vi "BioFeedback18(Producer+Consumer).vi"() -> ()   [LabVIEW 2016]
doc: "Use this template to build a producer/consumer design pattern. Use this template when you need to execute a process, such as data analysis, when a data source, such as a triggered acquisition, produces data at an uneven rate and you need to execute the process when the data becomes available."
uses:
  customSubVIs/8ChanWfmArray.ctl
  <vilib>/Waveform/WDTFileIO.llb/Export Waveforms To Spreadsheet File (1D).vi
panel:
  out "Disp Data":cluster{"queue out":refnum<queue>, dbl, dbl}[](array[cluster])
  in  "Target Percentage":dbl=10.0
  out "DisplayActivation":dbl
  out "DisplayBarActivation":dbl(slide) caption="Left" max=1.0 scale=0.0..100.0
  in  "Display Channel":dbl=0.5
  out "MVC Data":cluster{"queue out":refnum<queue>, dbl, dbl}[](array[cluster])
  in  "Base Name":string="Test"
  in  "Data Directory":path=path "C:/Users/Tinggroup/Desktop/VRMuscleActivationVisualizer/LabviewFiles/Data/Test"
  out "GetMaxStartTime":timestamp
  in  "MVC Number":dbl=1.0
  in  "SecondsToAcquireMax":dbl=3.0
  in  "Frames Per Second":dbl=30.0 caption="Upper Cut-Off"
  in  "EMG Input Device\nProduct Type":string="USB-6009"
  out "raw data":dynamicdata(graph)
  out "dispSize":dbl=20.0 caption="Lower Cut-Off"
  out "mvcSize":dbl=300.0 caption="Upper Cut-Off"
  in  "MVC Window Size (s)":dbl=0.5
  in  "Display Window Size (s)":dbl=0.5
  in  "MVC Raw Path":path
  in  "trial raw data":path
  in  "trial filtered data":path
  in  "MVC Filtered Path":path
  in  "Sample rate (Hz)":dbl=1000.0 caption="Upper Cut-Off"
  out "fps":dbl=20.0 caption="Lower Cut-Off"
  out "rate":dbl=300.0 caption="Upper Cut-Off"
  in  "Set Parameters":bool
  out "lower":dbl=20.0 caption="Lower Cut-Off"
  out "upper":dbl=300.0 caption="Upper Cut-Off"
  in  "Lower Cut-Off":dbl=20.0
  in  "Upper Cut-Off":dbl=500.0
  in  "Mark":bool
  in  "End Trial":bool
  in  "Reset MVC":bool
  in  "Get MVC":bool
  in  "StartTrial":bool
  out "State":T1(ring)
  out "FilteredAndRectified":waveform(dbl)[](graph) caption="Filtered and Rectified"
  in  "stop":bool
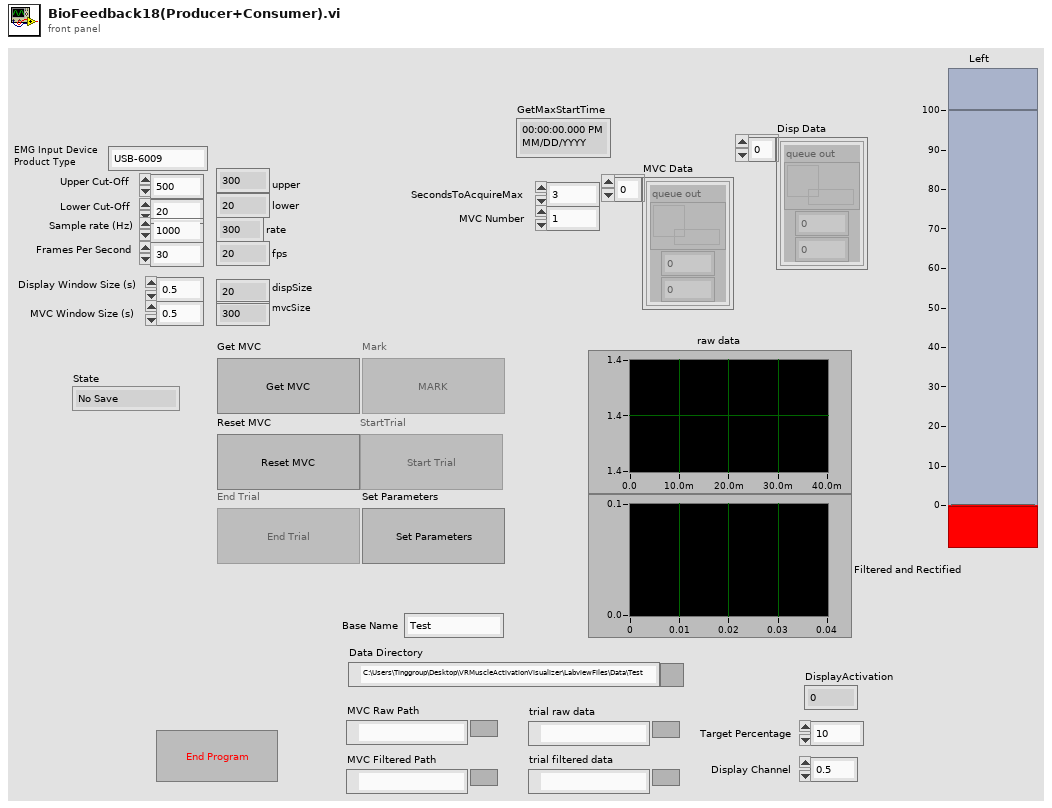
[diagram p1: front panel]
types:
  T1 = enum16{"No Save", "Acquiring Max", "Trial In Progress"}
  T2 = typedef "8ChanWfmArray.ctl" = waveform(dbl)[]
  T3 = enum8{"Enabled", "Disabled", "Disabled and Grayed Out"}
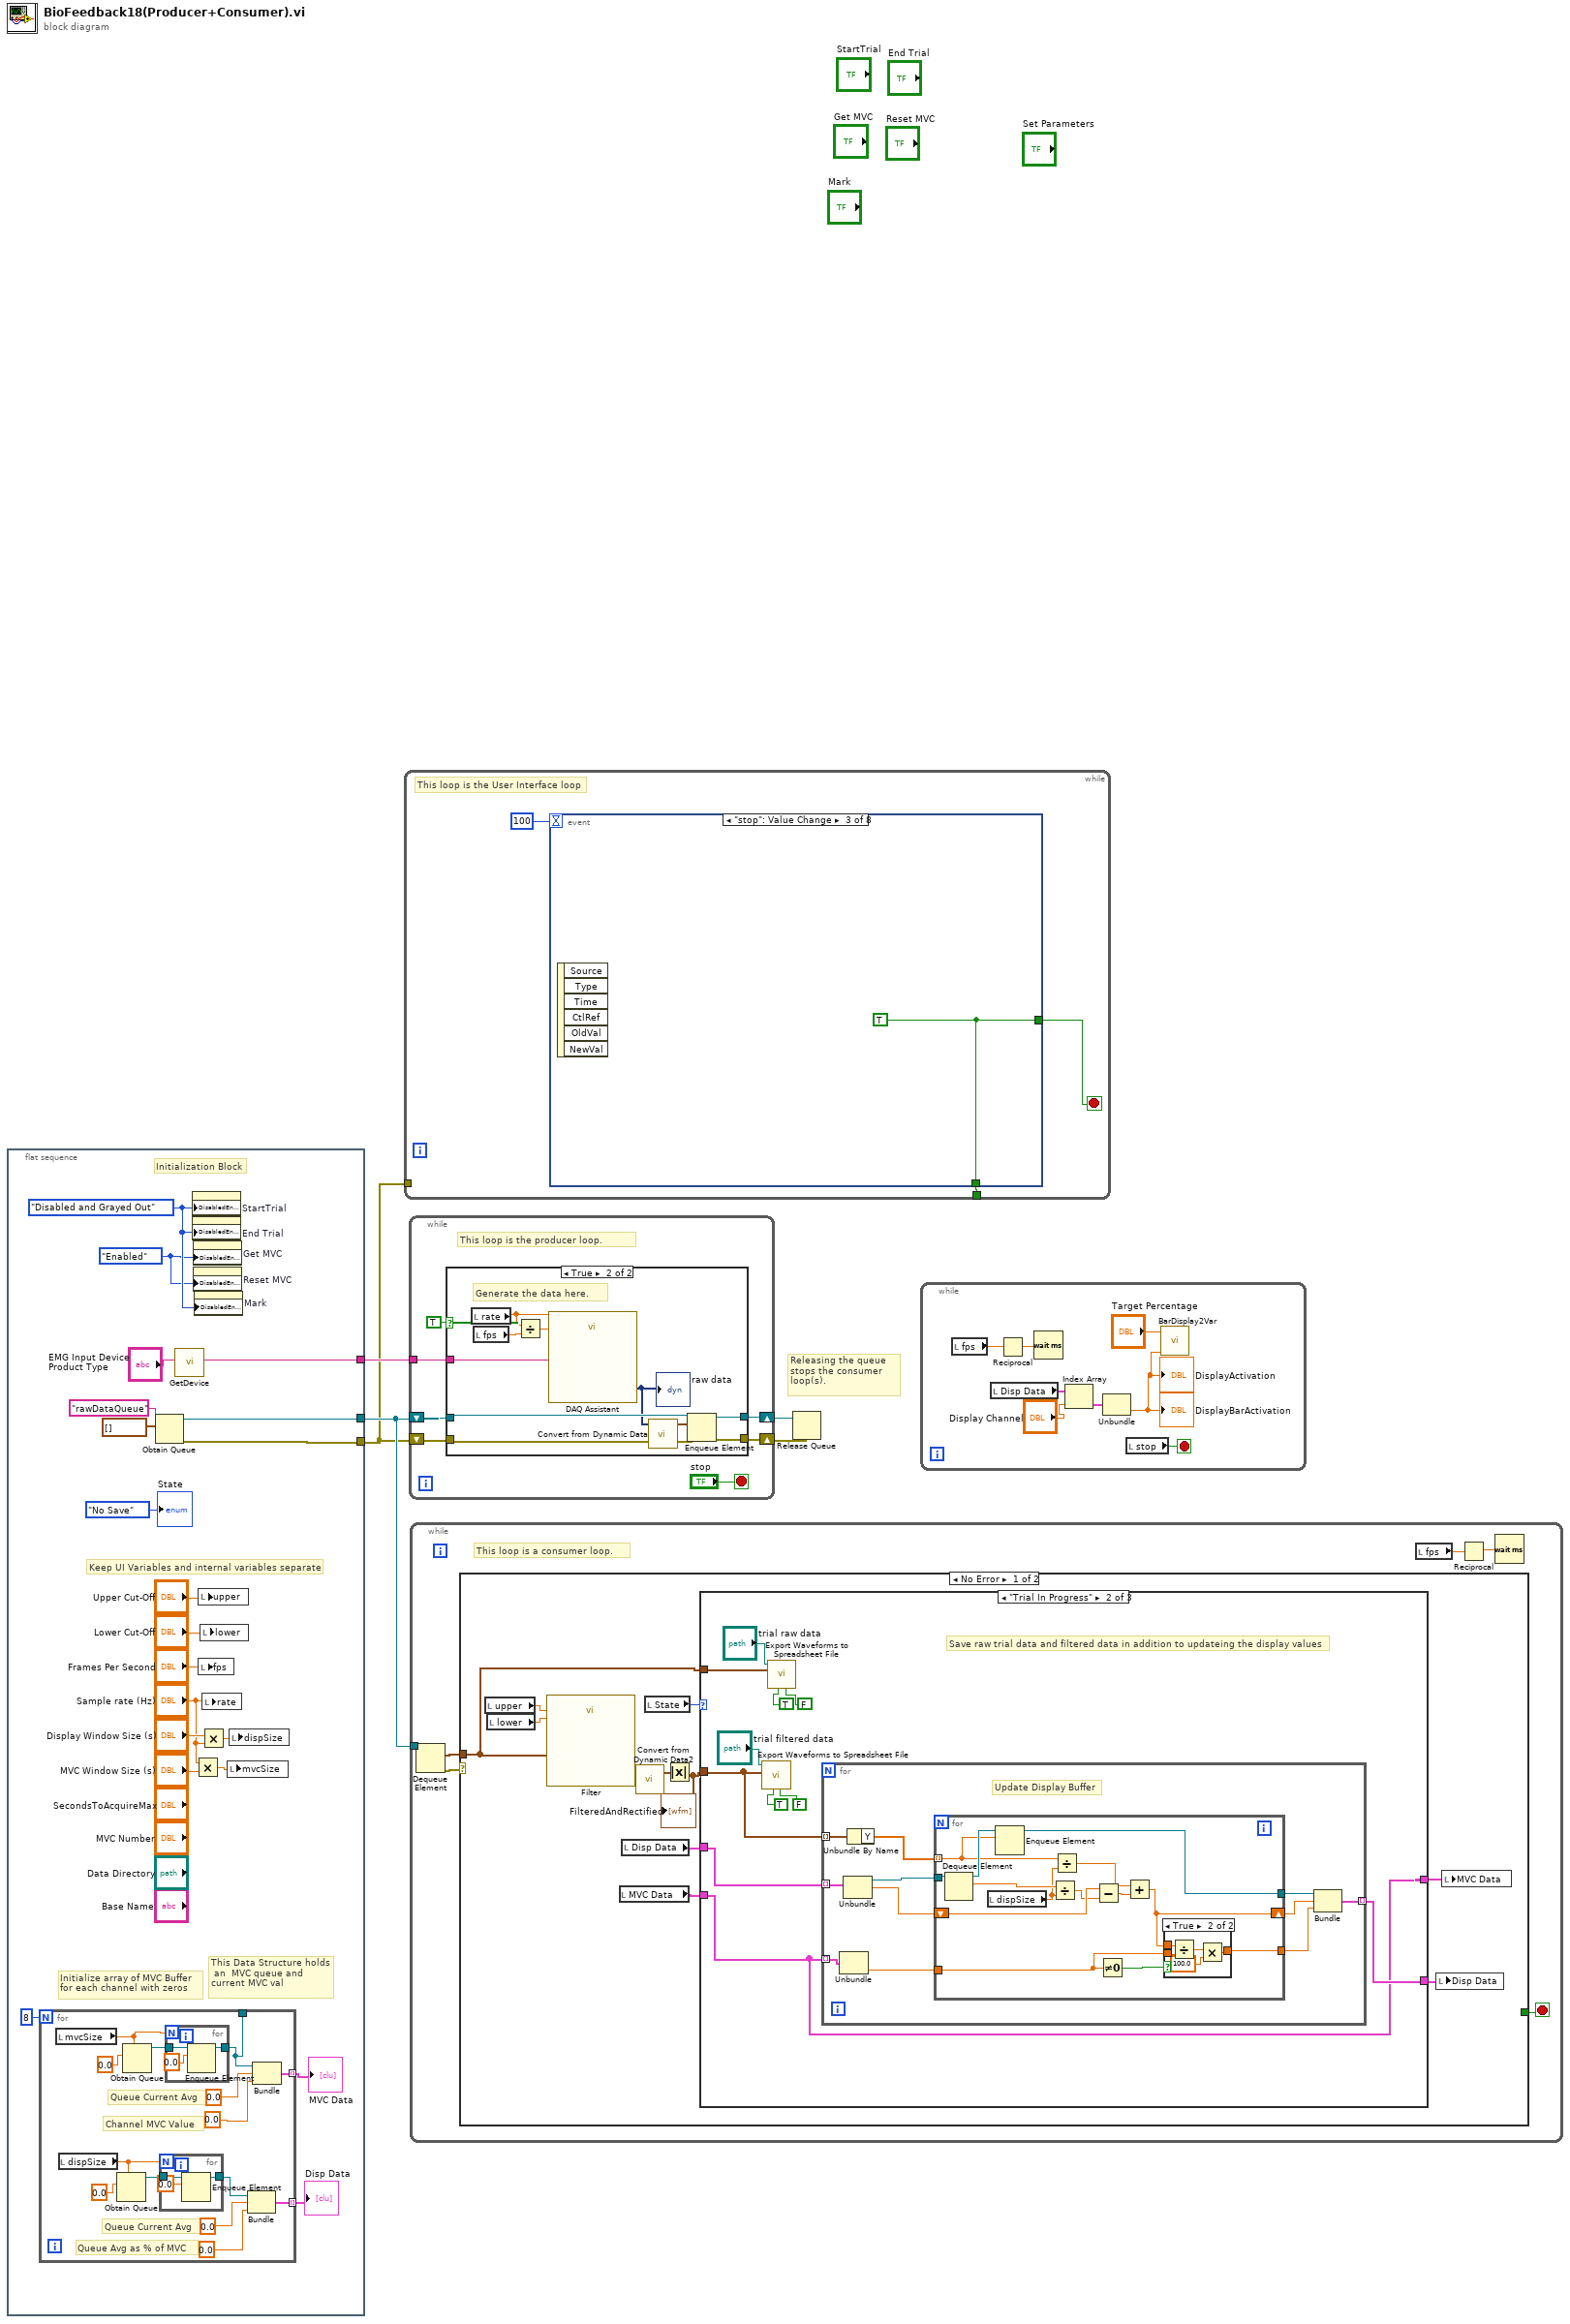
[diagram p0: block diagram]
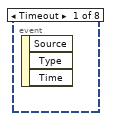
[diagram p2: hidden frame]
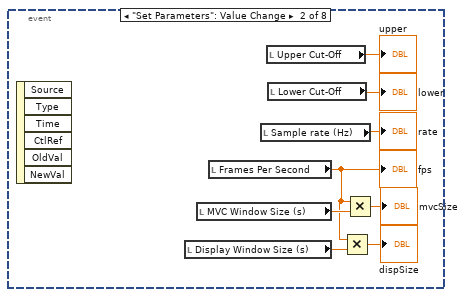
[diagram p3: hidden frame]
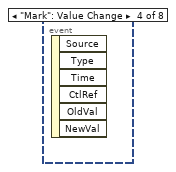
[diagram p4: hidden frame]
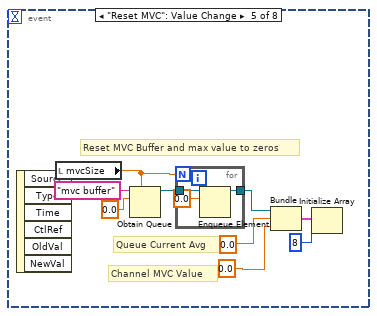
[diagram p5: hidden frame]
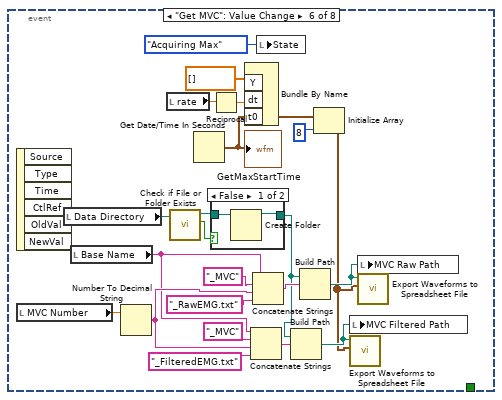
[diagram p6: hidden frame]
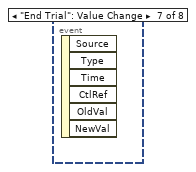
[diagram p8: hidden frame]
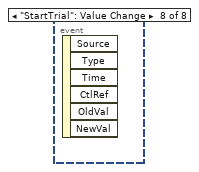
[diagram p9: hidden frame]
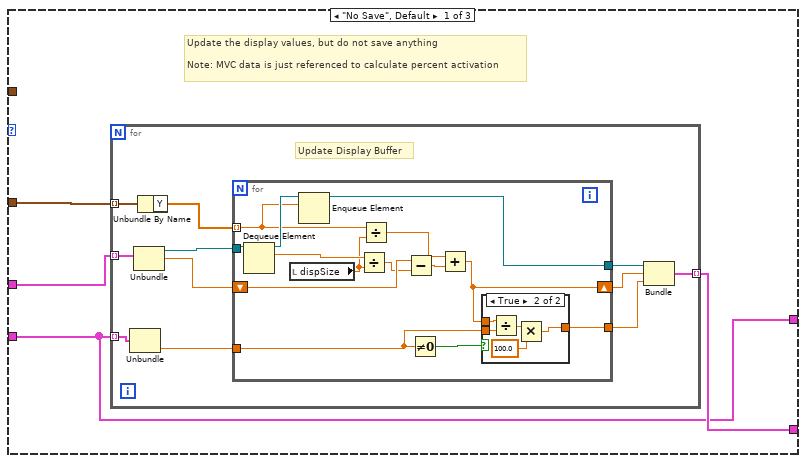
[diagram p10: hidden frame]
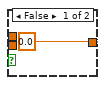
[diagram p11: hidden frame]
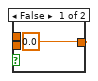
[diagram p12: hidden frame]
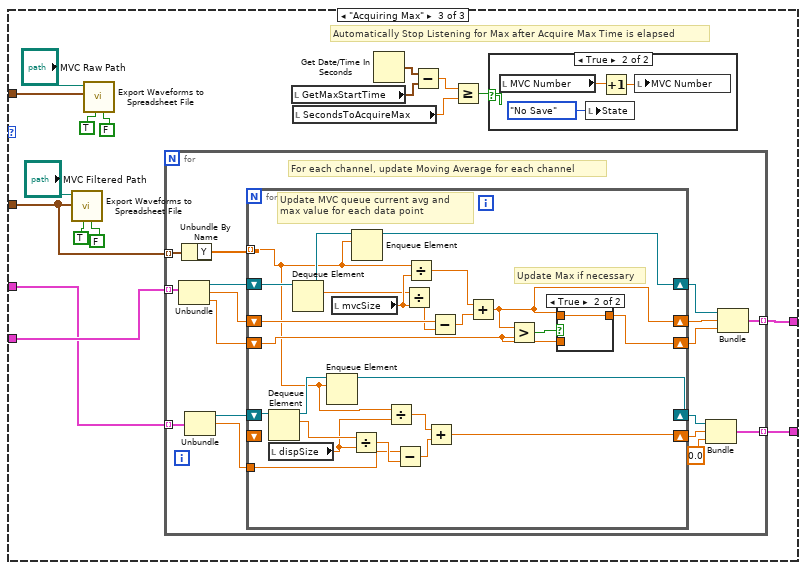
[diagram p13: hidden frame]
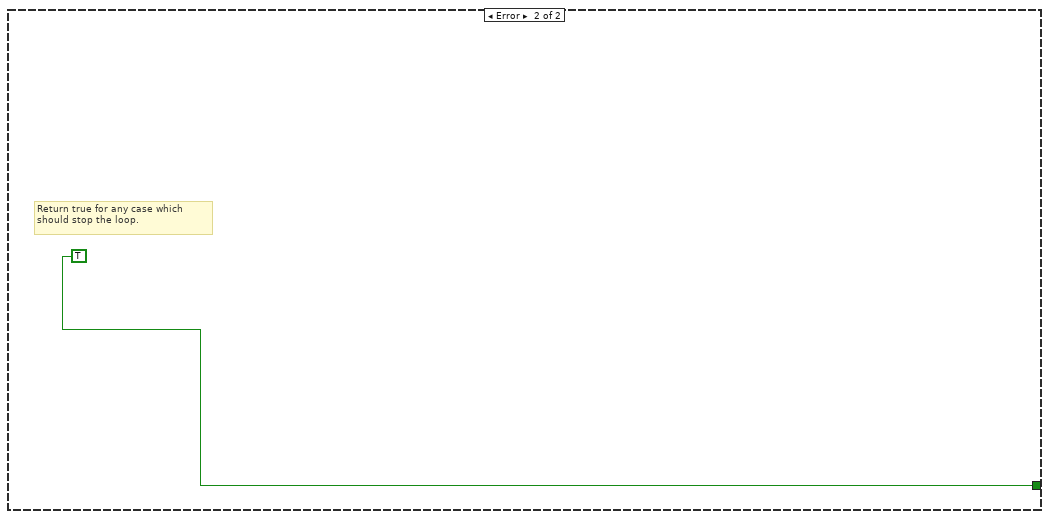
[diagram p16: hidden frame]
diagram:
  # "Releasing the queue stops the consumer loop(s)."
  n1 = flat-sequence {
    tunnel: [w16] -> w2
    tunnel: [w15] -> w1
    tunnel: [w18] -> w3
    frame #0 {
      w22 = T3."Enabled" ("Disabled")
      w23 = T3."Disabled and Grayed Out" ("Disabled")
      # "Keep UI Variables and internal variables separate"
      # "This Data Structure holds\n an  MVC queue and \ncurrent MVC val"
      # "Initialize array of MVC Buffer \nfor each channel with zeros"
      # "Initialization Block"
      n2 = for {
        N: 8 -> [_]
        tunnel: [w36] -> w8 mode=indexing
        tunnel: [w33] -> _
        tunnel: [w26] -> w7 mode=indexing
        # "Queue Avg as % of MVC"
        # "Queue Current Avg"
        # "Channel MVC Value"
        # "Queue Current Avg"
        n3 = local read "mvcSize"() -> (w37:dbl)
        n4 = local read "dispSize"() -> (w30:dbl)
        n5 = Obtain Queue(max queue size (-1, unlimited)=w30, element data type=0.0) -> (queue out=w27:refnum<queue>)  [unwired: 3 in, 2 out]
        n6 = Obtain Queue(max queue size (-1, unlimited)=w37, element data type=0.0) -> (queue out=w38:refnum<queue>)  [unwired: 3 in, 2 out]
        n7 = for {
          N: w30 -> [_]
          tunnel: w27 -> [w42]
          tunnel: [w40] -> w28
          n8 = Enqueue Element(queue=w42, element=0.0) -> (queue out=w40:refnum<queue>)  [unwired: 2 in, 2 out]
        }
        n9 = for {
          N: w37 -> [_]
          tunnel: w38 -> [w45]
          tunnel: [w43] -> w33
          n10 = Enqueue Element(queue=w45, element=0.0) -> (queue out=w43:refnum<queue>)  [unwired: 2 in, 2 out]
        }
        n11 = Bundle("queue out"=w28, 0.0, 0.0) -> (w26:cluster{"queue out":refnum<queue>, dbl, dbl})  [unwired: 1 in]
        n12 = Bundle("queue out"=w33, 0.0, 0.0) -> (w36:cluster{"queue out":refnum<queue>, dbl, dbl})  [unwired: 1 in]
      }
      "MVC Data" <- w8
      "Disp Data" <- w7
      n13 = Obtain Queue(name (unnamed)="rawDataQueue", element data type=T2 [] ("initialized array")) -> (queue out=w16:refnum<queue>, error out=w15:errorcluster)  [unwired: 3 in, 1 out]
      n14 = call "GetDevice.vi"("EMG Input Device\nProduct Type"="EMG Input Device\nProduct Type") -> ("DAQmx Device Name"=w18:tag)  [unwired: 10 in]
      n15 = property on="StartTrial" class="Bool"("DisabledEnum"=w23) -> ()  [unwired: 2 in, 2 out]
      n16 = property on="End Trial" class="Bool"("DisabledEnum"=w23) -> ()  [unwired: 2 in, 2 out]
      n17 = property on="Get MVC" class="Bool"("DisabledEnum"=w22) -> ()  [unwired: 2 in, 2 out]
      n18 = property on="Reset MVC" class="Bool"("DisabledEnum"=w22) -> ()  [unwired: 2 in, 2 out]
      n19 = property on="Mark" class="Bool"("DisabledEnum"=w23) -> ()  [unwired: 2 in, 2 out]
      n20 = Multiply(x="Sample rate (Hz)", y="MVC Window Size (s)") -> (x*y=w10:dbl)
      n21 = local write "upper"("Upper Cut-Off") -> ()
      n22 = local write "fps"("Frames Per Second") -> ()
      n23 = Multiply(x="Display Window Size (s)", y="Sample rate (Hz)") -> (x*y=w13:dbl)
      n24 = local write "lower"("Lower Cut-Off") -> ()
      n25 = local write "rate"("Sample rate (Hz)") -> ()
      n26 = local write "mvcSize"(w10) -> ()
      n27 = local write "dispSize"(w13) -> ()
      "State" <- T1."No Save" ("State")
    }
  }
  n28 = while {
    tunnel: [w47] -> _
    tunnel: w1 -> [_]
    stop <- w48 stop-if-true
    # "This loop is the User Interface loop"
    n29 = event shown="[2] \"stop\": Value Change" {
      selector: _ -> [_ _ _ _ _ _ _ _]
      dyn-events: _ -> [_ _ _ _ _ _ _ _]
      timeout: u32 100 ("milliseconds to wait") -> [_ _ _ _ _ _ _ _]
      tunnel: [_ _ w57 _ _ _ _ _] -> w48
      tunnel: [_ _ w57 _ _ _ _ _] -> w47
      event Timeout {
        n30 = event-data() -> ()  [unwired: 1 in, 3 out]
      }
      event "Set Parameters": Value Change {
        n31 = event-data() -> ()  [unwired: 1 in, 6 out]
        n32 = local read "Display Window Size (s)"() -> (w52:dbl)
        n33 = local read "MVC Window Size (s)"() -> (w53:dbl)
        n34 = local read "Frames Per Second"() -> (w51:dbl)
        "fps" <- w51
        n35 = local read "Sample rate (Hz)"() -> (→"rate":dbl)
        n36 = local read "Upper Cut-Off"() -> (→"upper":dbl)
        n37 = local read "Lower Cut-Off"() -> (→"lower":dbl)
        n38 = Multiply(x=w51, y=w52) -> (x*y=→"dispSize":dbl)
        n39 = Multiply(x=w51, y=w53) -> (x*y=→"mvcSize":dbl)
      }
      event "stop": Value Change {
        w57 = TRUE
        n40 = event-data() -> ()  [unwired: 1 in, 6 out]
      }
      event "Mark": Value Change {
        n41 = event-data() -> ()  [unwired: 1 in, 6 out]
      }
      event "Reset MVC": Value Change {
        # "Channel MVC Value"
        # "Queue Current Avg"
        # "Reset MVC Buffer and max value to zeros"
        n42 = event-data() -> ()  [unwired: 1 in, 6 out]
        n43 = local read "mvcSize"() -> (w61:dbl)
        n44 = Obtain Queue(max queue size (-1, unlimited)=w61, name (unnamed)="mvc buffer", element data type=0.0) -> (queue out=w60:refnum<queue>)  [unwired: 2 in, 2 out]
        n45 = for {
          N: w61 -> [_]
          tunnel: w60 -> [w69]
          tunnel: [w67] -> w63
          n46 = Enqueue Element(queue=w69, element=0.0) -> (queue out=w67:refnum<queue>)  [unwired: 2 in, 2 out]
        }
        n47 = Bundle("queue out"=w63, 0.0, 0.0) -> (w64:cluster{"queue out":refnum<queue>, dbl, dbl})  [unwired: 1 in]
        n48 = Initialize Array(w64, 8 ("dimension size")) -> ()  [unwired: 1 out]
      }
      event "Get MVC": Value Change {
        n49 = event-data() -> ()  [unwired: 1 in, 6 out]
        n50 = local read "MVC Number"() -> (w79:dbl)
        n51 = local read "Data Directory"() -> (w80:path)
        n52 = local read "Base Name"() -> (w77:string)
        n53 = Number To Decimal String(number=w79) -> (decimal integer string=w78:string)  [unwired: 1 in]
        n54 = local read "rate"() -> (w74:dbl)
        n55 = call <vilib>:"Check if File or Folder Exists.vi"("path"=w80) -> ("file or folder exists?"=w82:bool, "dup path"=w81:path)  [unwired: 8 in, 1 out]
        n56 = Get Date/Time In Seconds() -> (seconds since 1Jan1904=w70:timestamp)
        "GetMaxStartTime" <- w70
        n57 = Reciprocal(x=w74) -> (1/x=w73:dbl)
        n58 = case shown="False" w82 {
          tunnel: w81 -> [w94 w95]
          tunnel: [w93 w95] -> w83
          frame False {
            n59 = Create Folder(path (use dialog)=w94) -> (created path=w93:path)  [unwired: 2 in, 2 out]
          }
          frame True {
          }
        }
        n60 = Bundle By Name("Y"=dbl[] [], "dt"=w73, "t0"=w70) -> (w76:waveform(dbl))  [unwired: 1 in]
        n61 = Concatenate Strings(w77, "_MVC" ("string"), w78, "_FilteredEMG.txt" ("string")) -> (w90:string)
        n62 = Concatenate Strings(w77, "_MVC" ("string"), w78, "_RawEMG.txt" ("string")) -> (w89:string)
        n63 = local write "State"(T1."Acquiring Max" ("State")) -> ()
        n64 = Build Path(base path=w83, name or relative path=w90) -> (appended path=w84:path)
        n65 = Build Path(base path=w83, name or relative path=w89) -> (appended path=w85:path)
        n66 = Initialize Array(w76, 8 ("dimension size")) -> (w75:waveform(dbl)[])
        n67 = local write "MVC Filtered Path"(w84) -> ()
        n68 = call-poly <vilib>:"Export Waveforms to Spreadsheet File.vi"("waveforms"=w75, "file path (dialog if empty)"=w84) -> ()  [unwired: 8 in, 2 out]
        n69 = local write "MVC Raw Path"(w85) -> ()
        n70 = call-poly <vilib>:"Export Waveforms to Spreadsheet File.vi"("waveforms"=w75, "file path (dialog if empty)"=w85) -> ()  [unwired: 8 in, 2 out]
      }
      event "End Trial": Value Change {
        n71 = event-data() -> ()  [unwired: 1 in, 6 out]
      }
      event "StartTrial": Value Change {
        n72 = event-data() -> ()  [unwired: 1 in, 6 out]
      }
    }
  }
  n73 = while {
    shift-right: [w98] -> w4
    shift-left: w1 -> [w99]
    shift-right: [w100] -> w5
    shift-left: w2 -> [w101]
    tunnel: w3 -> [w96]
    stop <- "stop" stop-if-true
    # "This loop is the producer loop."
    n74 = case shown="True" TRUE ("Case Constant\n(See Context Help)") {
      tunnel: w101 -> [w104 w114]
      tunnel: [w104 w113] -> w100
      tunnel: w99 -> [w103 w112]
      tunnel: [w103 w111] -> w98
      tunnel: w96 -> [_ w105]
      frame False {
      }
      frame True {
        # "Generate the data here."
        n75 = local read "rate"() -> (w108:dbl)
        n76 = local read "fps"() -> (w109:dbl)
        n77 = Divide(x=w108, y=w109) -> (x/y=w107:dbl)
        n78 = call "DAQ Assistant"("rate"=w108, "number of samples"=w107, "device name"=w105) -> ("data"=w106:dynamicdata)  [unwired: 13 in, 3 out]
        "raw data" <- w106
        n79 = call "Convert from Dynamic Data"("Dynamic Data Type"=w106) -> ("Array of Waveform"=w110:waveform(dbl)[])  [unwired: 3 in]
        n80 = Enqueue Element(queue=w114, element=w110, error in (no error)=w112) -> (queue out=w113:refnum<queue>, error out=w111:errorcluster)  [unwired: 1 in, 1 out]
      }
    }
  }
  n81 = while {
    tunnel: w2 -> [w117]
    stop <- w118 stop-if-true
    # "This loop is a consumer loop."
    n82 = Dequeue Element(queue=w117) -> (element=w119:T2, error out=w120:errorcluster)  [unwired: 2 in, 2 out]
    n83 = case shown="No Error" w120 {
      tunnel: w119 -> [w126 _]
      tunnel: [_ TRUE] -> w118
      frame No Error {
        n84 = local read "upper"() -> (w129:dbl)
        n85 = local read "lower"() -> (w128:dbl)
        n86 = call "Filter"("Lower Cut-Off"=w128, "Upper Cut-Off"=w129, "Signal"=w126) -> ("Filtered Signal"=w130:dynamicdata)  [unwired: 7 in, 1 out]
        n87 = local read "MVC Data"() -> (w124:cluster{"queue out":refnum<queue>, dbl, dbl}[])
        n88 = local read "Disp Data"() -> (w123:cluster{"queue out":refnum<queue>, dbl, dbl}[])
        n89 = call "Convert from Dynamic Data2"("Dynamic Data Type"=w130) -> ("Array of Waveform"=w131:waveform(dbl)[])  [unwired: 3 in]
        n90 = local read "State"() -> (w127:T1)
        n91 = Absolute Value(x=w131) -> (abs(x)=w125:waveform(dbl)[])
        "FilteredAndRectified" <- w125
        n92 = case shown="\"Trial In Progress\"" w127 {
          tunnel: w125 -> [w135 w169 w219]
          tunnel: w126 -> [_ w172 w220]
          tunnel: w124 -> [w132 w167 w210]
          tunnel: w123 -> [w134 w170 w209]
          tunnel: [w133 w168 w211] -> w121
          tunnel: [w132 w167 w212] -> w122
          frame "No Save", Default {
            # "Update the display values, but do not save anything\n\nNote: MVC data is just referenced to calculate percent activation"
            n93 = for {
              tunnel: w134 -> [w140] mode=indexing
              tunnel: w135 -> [w145] mode=indexing
              tunnel: [w141] -> w133 mode=indexing
              tunnel: w132 -> [w138] mode=indexing
              # "Update Display Buffer"
              n94 = Unbundle(w138) -> (w137:dbl)  [unwired: 2 out]
              n95 = Unbundle(w140) -> ("queue out"=w146:refnum<queue>, w139:dbl)  [unwired: 1 out]
              n96 = Unbundle By Name(w145) -> ("Y"=w144:dbl[])
              n97 = for {
                tunnel: w146 -> [w154]
                tunnel: w144 -> [w150] mode=indexing
                shift-right: [w148] -> w143
                shift-left: w139 -> [w159]
                tunnel: [w149] -> w142
                tunnel: w137 -> [w152]
                tunnel: [w147] -> w136
                n98 = Dequeue Element(queue=w154) -> (queue out=w151:refnum<queue>, element=w160:dbl)  [unwired: 2 in, 2 out]
                n99 = local read "dispSize"() -> (w157:dbl)
                n100 = Enqueue Element(queue=w151, element=w150) -> (queue out=w149:refnum<queue>)  [unwired: 2 in, 2 out]
                n101 = Divide(x=w160, y=w157) -> (x/y=w158:dbl)
                n102 = Divide(x=w150, y=w157) -> (x/y=w155:dbl)
                n103 = Subtract(x=w159, y=w158) -> (x-y=w156:dbl)
                n104 = Not Equal To 0?(x=w152) -> (x != 0?=w153:bool)
                n105 = Add(x=w155, y=w156) -> (x+y=w148:dbl)
                n106 = case shown="True" w153 {
                  tunnel: w152 -> [_ w166]
                  tunnel: [0.0 w162] -> w147
                  tunnel: w148 -> [_ w165]
                  frame False {
                  }
                  frame True {
                    n107 = Divide(x=w165, y=w166) -> (x/y=w163:dbl)
                    n108 = Multiply(x=w163, y=100.0) -> (x*y=w162:dbl)
                  }
                }
              }
              n109 = Bundle("queue out"=w142, w143, w136) -> (w141:cluster{"queue out":refnum<queue>, dbl, dbl})  [unwired: 1 in]
            }
          }
          frame "Trial In Progress" {
            # "Save raw trial data and filtered data in addition to updateing the display values"
            n110 = call-poly <vilib>:"Export Waveforms to Spreadsheet File.vi"("header? (write header:T)"=FALSE, "append to file? (new file:F)"=TRUE, "waveforms"=w169, "file path (dialog if empty)"="trial filtered data") -> ()  [unwired: 6 in, 2 out]
            n111 = call-poly <vilib>:"Export Waveforms to Spreadsheet File.vi"("header? (write header:T)"=FALSE, "append to file? (new file:F)"=TRUE, "waveforms"=w172, "file path (dialog if empty)"="trial raw data") -> ()  [unwired: 6 in, 2 out]
            n112 = for {
              tunnel: w170 -> [w182] mode=indexing
              tunnel: w169 -> [w187] mode=indexing
              tunnel: [w183] -> w168 mode=indexing
              tunnel: w167 -> [w180] mode=indexing
              # "Update Display Buffer"
              n113 = Unbundle(w180) -> (w179:dbl)  [unwired: 2 out]
              n114 = Unbundle(w182) -> ("queue out"=w188:refnum<queue>, w181:dbl)  [unwired: 1 out]
              n115 = Unbundle By Name(w187) -> ("Y"=w186:dbl[])
              n116 = for {
                tunnel: w188 -> [w196]
                tunnel: w186 -> [w192] mode=indexing
                shift-right: [w190] -> w185
                shift-left: w181 -> [w201]
                tunnel: [w191] -> w184
                tunnel: w179 -> [w194]
                tunnel: [w189] -> w178
                n117 = Dequeue Element(queue=w196) -> (queue out=w193:refnum<queue>, element=w202:dbl)  [unwired: 2 in, 2 out]
                n118 = local read "dispSize"() -> (w199:dbl)
                n119 = Enqueue Element(queue=w193, element=w192) -> (queue out=w191:refnum<queue>)  [unwired: 2 in, 2 out]
                n120 = Divide(x=w202, y=w199) -> (x/y=w200:dbl)
                n121 = Divide(x=w192, y=w199) -> (x/y=w197:dbl)
                n122 = Subtract(x=w201, y=w200) -> (x-y=w198:dbl)
                n123 = Not Equal To 0?(x=w194) -> (x != 0?=w195:bool)
                n124 = Add(x=w197, y=w198) -> (x+y=w190:dbl)
                n125 = case shown="True" w195 {
                  tunnel: w194 -> [_ w208]
                  tunnel: [0.0 w206] -> w189
                  tunnel: w190 -> [_ w207]
                  frame False {
                  }
                  frame True {
                    n126 = Divide(x=w207, y=w208) -> (x/y=w205:dbl)
                    n127 = Multiply(x=w205, y=100.0) -> (x*y=w206:dbl)
                  }
                }
              }
              n128 = Bundle("queue out"=w184, w185, w178) -> (w183:cluster{"queue out":refnum<queue>, dbl, dbl})  [unwired: 1 in]
            }
          }
          frame "Acquiring Max" {
            # "Automatically Stop Listening for Max after Acquire Max Time is elapsed"
            n129 = call-poly <vilib>:"Export Waveforms to Spreadsheet File.vi"("header? (write header:T)"=FALSE, "append to file? (new file:F)"=TRUE, "waveforms"=w219, "file path (dialog if empty)"="MVC Filtered Path") -> ()  [unwired: 6 in, 2 out]
            n130 = call-poly <vilib>:"Export Waveforms to Spreadsheet File.vi"("header? (write header:T)"=FALSE, "append to file? (new file:F)"=TRUE, "waveforms"=w220, "file path (dialog if empty)"="MVC Raw Path") -> ()  [unwired: 6 in, 2 out]
            n131 = for {
              tunnel: w219 -> [w245] mode=indexing
              tunnel: w210 -> [w243] mode=indexing
              tunnel: [w237] -> w212 mode=indexing
              tunnel: w209 -> [w235] mode=indexing
              tunnel: [w229] -> w211 mode=indexing
              # "For each channel, update Moving Average for each channel"
              n132 = Unbundle(w243) -> ("queue out"=w236:refnum<queue>, w242:dbl, w241:dbl)
              n133 = Unbundle By Name(w245) -> ("Y"=w244:dbl[])
              n134 = Unbundle(w235) -> ("queue out"=w231:refnum<queue>, w234:dbl)  [unwired: 1 out]
              n135 = for {
                tunnel: w244 -> [w252] mode=indexing
                shift-right: [w257] -> w239
                shift-left: w242 -> [w269]
                shift-right: [w261] -> w240
                shift-left: w236 -> [w260]
                shift-right: [w263] -> w238
                shift-left: w241 -> [w262]
                tunnel: w234 -> [w250]
                shift-right: [w247] -> w232
                shift-left: _ -> [_]
                shift-right: [w254] -> w233
                shift-left: w231 -> [w246]
                # "Update Max if necessary"
                # "Update MVC queue current avg and \nmax value for each data point"
                n136 = Dequeue Element(queue=w246) -> (queue out=w256:refnum<queue>, element=w255:dbl)  [unwired: 2 in, 2 out]
                n137 = local read "dispSize"() -> (w253:dbl)
                n138 = Dequeue Element(queue=w260) -> (queue out=w259:refnum<queue>, element=w258:dbl)  [unwired: 2 in, 2 out]
                n139 = Enqueue Element(queue=w256, element=w252) -> (queue out=w254:refnum<queue>)  [unwired: 2 in, 2 out]
                n140 = local read "mvcSize"() -> (w267:dbl)
                n141 = Divide(x=w255, y=w253) -> (x/y=w251:dbl)
                n142 = Enqueue Element(queue=w259, element=w252) -> (queue out=w261:refnum<queue>)  [unwired: 2 in, 2 out]
                n143 = Divide(x=w252, y=w253) -> (x/y=w249:dbl)
                n144 = Subtract(x=w250, y=w251) -> (x-y=w248:dbl)
                n145 = Divide(x=w258, y=w267) -> (x/y=w268:dbl)
                n146 = Divide(x=w252, y=w267) -> (x/y=w265:dbl)
                n147 = Add(x=w249, y=w248) -> (x+y=w247:dbl)
                n148 = Subtract(x=w269, y=w268) -> (x-y=w266:dbl)
                n149 = Add(x=w265, y=w266) -> (x+y=w257:dbl)
                n150 = Greater?(x=w257, y=w262) -> (0:w264:bool)
                n151 = case shown="True" w264 {
                  tunnel: w257 -> [_ w271]
                  tunnel: [w270 w271] -> w263
                  tunnel: w262 -> [w270 _]
                  frame False {
                  }
                  frame True {
                  }
                }
              }
              n152 = Bundle("queue out"=w233, w232, 0.0) -> (w229:cluster{"queue out":refnum<queue>, dbl, dbl})  [unwired: 1 in]
              n153 = Bundle("queue out"=w240, w239, w238) -> (w237:cluster{"queue out":refnum<queue>, dbl, dbl})  [unwired: 1 in]
            }
            n154 = local read "GetMaxStartTime"() -> (w216:timestamp)
            n155 = local read "SecondsToAcquireMax"() -> (w214:dbl)
            n156 = Get Date/Time In Seconds() -> (seconds since 1Jan1904=w217:timestamp)
            n157 = Subtract(x=w217, y=w216) -> (x-y=w215:dbl)
            n158 = Greater Or Equal?(x=w215, y=w214) -> (x >= y?=w213:bool)
            n159 = case shown="True" w213 {
              frame False {
              }
              frame True {
                n160 = local read "MVC Number"() -> (w228:dbl)
                n161 = local write "State"(T1."No Save" ("State")) -> ()
                n162 = Increment(x=w228) -> (x+1=w227:dbl)
                n163 = local write "MVC Number"(w227) -> ()
              }
            }
          }
        }
        n164 = local write "Disp Data"(w121) -> ()
        n165 = local write "MVC Data"(w122) -> ()
      }
      frame Error {
        # "Return true for any case which should stop the loop."
      }
    }
    n166 = local read "fps"() -> (w115:dbl)
    n167 = Reciprocal(x=w115) -> (1/x=w116:dbl)
    n168 = Wait (ms)(milliseconds to wait=w116) -> ()  [unwired: 1 out]
  }
  n169 = Release Queue(queue=w5, error in (no error)=w4) -> ()  [unwired: 1 in, 3 out]
  n170 = while {
    stop <- w273 stop-if-true
    n171 = local read "fps"() -> (w275:dbl)
    n172 = local read "Disp Data"() -> (w279:cluster{"queue out":refnum<queue>, dbl, dbl}[])
    n173 = Reciprocal(x=w275) -> (1/x=w274:dbl)
    n174 = Wait (ms)(milliseconds to wait=w274) -> ()  [unwired: 1 out]
    n175 = Index Array(array=w279, index="Display Channel") -> (element=w277:cluster{"queue out":refnum<queue>, dbl, dbl})
    n176 = Unbundle(w277) -> (w276:dbl)  [unwired: 2 out]
    "DisplayBarActivation" <- w276
    "DisplayActivation" <- w276
    n177 = local read "stop"() -> (w273:bool)
    n178 = call "BarDisplay2Var.vi"("Activation Percentage"=w276, "Target Percentage"="Target Percentage") -> ()  [unwired: 10 in]
  }
